vi "Heater Status.vi"(8 "error in (no error)":errorcluster, 10 "Heater Output (1:1)":u16(ring)=1 items=["1"=1, "2"=2], 11 "VISA resource name":refnum<visa-resource-name>) -> (0 "error out":errorcluster, 1 "Heater Range":u16(ring) items=["Off", "Low (On)", "Medium", "High"], 2 "Heater Status":u16(ring) items=["No Error", "Heater Open Load", "Heater Short"], 3 "VISA resource name out":refnum<visa-resource-name>, 4 "Manual Output Value":dbl format="%.2f")   [LabVIEW 2014, in "Lake Shore 335.lvlib"]
doc: "Returns the Heater Output status, Manual Output value, and Heater Range. The output will be turned off in the event of an open or short circuit error condition. An error condition is cleared upon querying the heater status, which will also clear the front panel error message."
uses:
  Lake Shore 335.lvlib
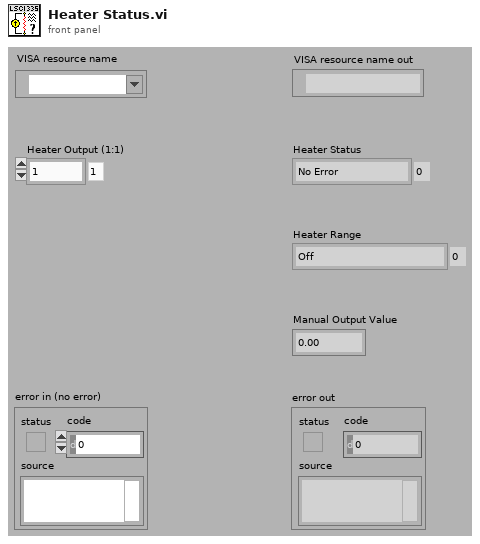
[diagram p1: front panel]
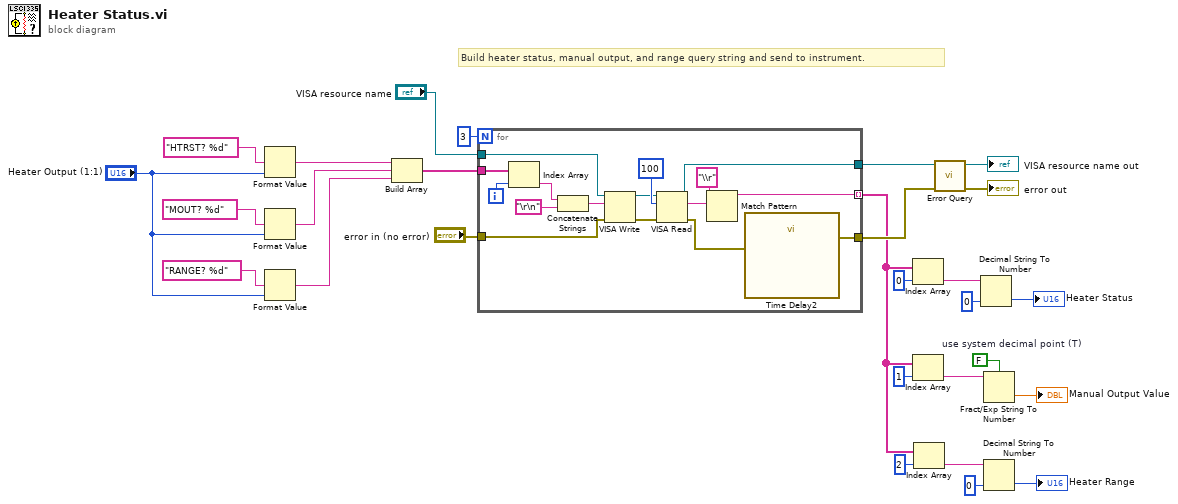
[diagram p0: block diagram]
diagram:
  w8 = FALSE  # use system decimal point (T)
  # "Build heater status, manual output, and range query string and send to instrument."
  n1 = Format Value(format string="HTRST? %d", value (0)="Heater Output (1:1)") -> (output string=w20:string)  [unwired: 1 in]
  n2 = Format Value(format string="MOUT? %d", value (0)="Heater Output (1:1)") -> (output string=w10:string)  [unwired: 1 in]
  n3 = Format Value(format string="RANGE? %d", value (0)="Heater Output (1:1)") -> (output string=w9:string)  [unwired: 1 in]
  n4 = Build Array(w20, w10, w9) -> (w23:string[])
  n5 = for {
    N: 3 -> [_]
    tunnel: [w38] -> w15
    tunnel: [w32] -> w14
    tunnel: "VISA resource name" -> [w37]
    tunnel: "error in (no error)" -> [w36]
    tunnel: w23 -> [w35]
    tunnel: [w34] -> w4 mode=indexing
    i -> [w39]
    n6 = Index Array(array=w35, index=w39) -> (element=w30:string)
    n7 = Concatenate Strings(w30, "\r\n") -> (w31:string)
    n8 = VISA Write(VISA resource name=w37, write buffer=w31, error in (no error)=w36) -> (VISA resource name out=w41:refnum<visa-resource-name>, error out=w40:errorcluster)  [unwired: 1 out]
    n9 = VISA Read(VISA resource name=w41, byte count=100, error in (no error)=w40) -> (VISA resource name out=w38:refnum<visa-resource-name>, read buffer=w43:string, error out=w33:errorcluster)  [unwired: 1 out]
    n10 = Match Pattern(string=w43, regular expression="\\r") -> (before substring=w34:string)  [unwired: 1 in, 3 out]
    n11 = call "Time Delay2"("error in (no error)"=w33) -> ("error out"=w32:errorcluster)  [unwired: 10 in]
  }
  n12 = Index Array(array=w4, index=0) -> (element=w19:string)
  n13 = Index Array(array=w4, index=1) -> (element=w7:string)
  n14 = Index Array(array=w4, index=2) -> (element=w2:string)
  n15 = call "Error Query.vi"("error in (no error)"=w14, "VISA resource name"=w15) -> ("error out"=→"error out":errorcluster, "VISA resource name out"=→"VISA resource name out":refnum<visa-resource-name>)  [unwired: 7 in, 1 out]
  n16 = Decimal String To Number(string=w19, default (0L)=u16 0) -> (number=→"Heater Status":u16)  [unwired: 1 in, 1 out]
  n17 = Fract/Exp String To Number(use system decimal point (T)=w8, string=w7) -> (number=→"Manual Output Value":dbl)  [unwired: 2 in, 1 out]
  n18 = Decimal String To Number(string=w2, default (0L)=u16 0) -> (number=→"Heater Range":u16)  [unwired: 1 in, 1 out]
